vi "Get Queue Index for Resource.vi"(10 "Resource":string, 11 "Communication Configuration":T1) -> (3 "Index":i32)   [LabVIEW 2017, in "Routing and Faulting Engine.lvlib"]
uses:
  Routing and Faulting Engine.lvlib
  Shared/Communication Configuration.ctl
  Shared/Routing and Faulting Shared.lvlib
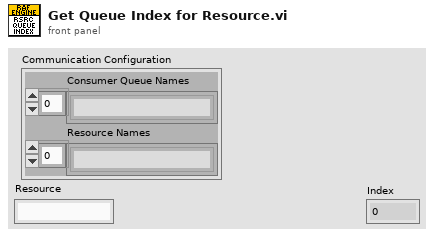
[diagram p1: front panel]
types:
  T1 = typedef "Routing and Faulting Shared.lvlib/Communication Configuration.ctl" = cluster{"Consumer Queue Names":string[], "Resource Names":string[]}
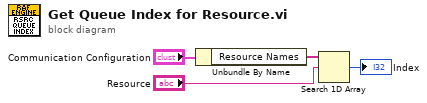
[diagram p0: block diagram]
diagram:
  n1 = Unbundle By Name("Communication Configuration") -> ("Resource Names"=w3:string[])
  n2 = Search 1D Array(1D array=w3, element="Resource") -> (index of element=→"Index":i32)  [unwired: 1 in]
